vi "Set-control-enable.vi"   [LabVIEW 2013, in "MaterialCharacterization.lvlib" / "MC-UI.lvclass"]
uses:
  MC-UI.lvclass
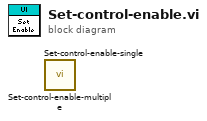
[diagram p0: block diagram]
diagram:
  n1 = call "Set-control-enable-multiple.vi"() -> ()  [unwired: 10 in, 2 out]
  n2 = call "Set-control-enable-single.vi"() -> ()  [unwired: 10 in, 2 out]
